vi "Scanner_Ansteuerung_Prepare_Puls_Sequence.vi"(11 "cluster":T1) -> (0 "Sync-Pulse-Array":bool[](array[boolean]), 1 "Power-Array":dbl[][][](array[numeric]), 3 "Clock-Array":i32[](array[numeric]))   [LabVIEW 2009]
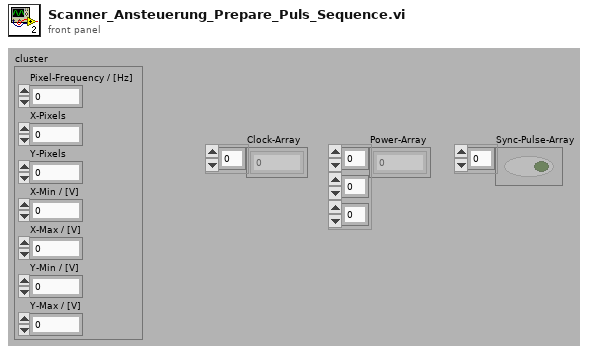
[diagram p1: front panel]
types:
  T1 = cluster{"Pixel-Frequency / [Hz]":dbl, "X-Pixels":u32, "Y-Pixels":u32, "X-Min / [V]":dbl, "X-Max / [V]":dbl, "Y-Min / [V]":dbl, "Y-Max / [V]":dbl}
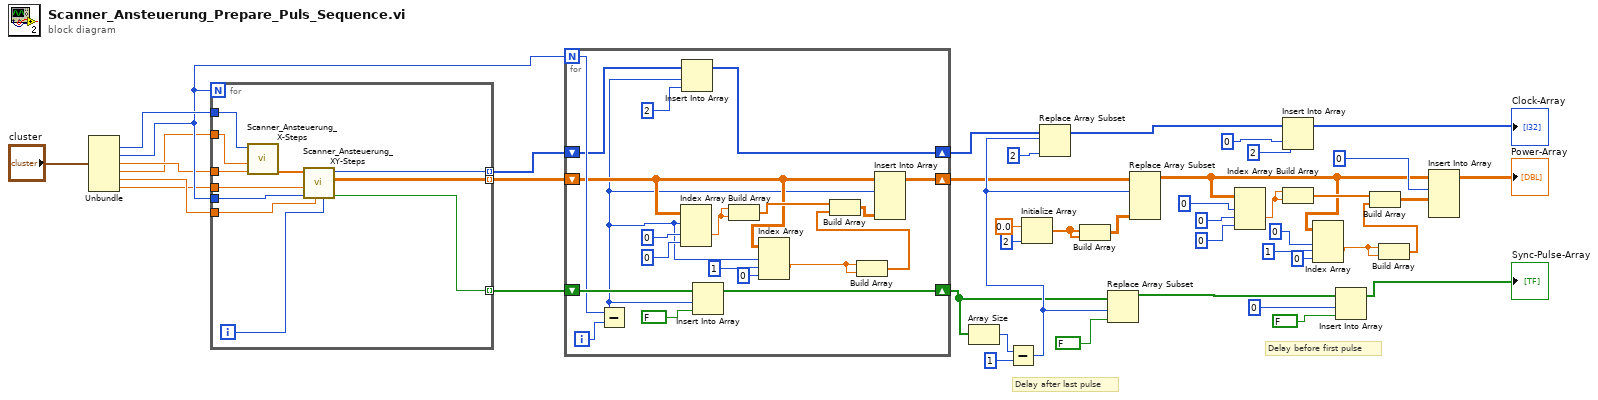
[diagram p0: block diagram]
diagram:
  # "Delay before first pulse"
  # "Delay after last pulse"
  n1 = Unbundle("cluster") -> ("X-Pixels"=w6:u32, "Y-Pixels"=w5:u32, "X-Min / [V]"=w4:dbl, "X-Max / [V]"=w3:dbl, "Y-Min / [V]"=w2:dbl, "Y-Max / [V]"=w1:dbl)  [unwired: 1 out]
  n2 = for {
    N: w5 -> [_]
    tunnel: w2 -> [w55]
    tunnel: w4 -> [w54]
    tunnel: w6 -> [w53]
    tunnel: w3 -> [w52]
    tunnel: w1 -> [w51]
    tunnel: w5 -> [w50]
    tunnel: [w49] -> w9 mode=indexing
    tunnel: [w47] -> w8 mode=indexing
    tunnel: [w46] -> w10 mode=indexing
    i -> [w45]
    n3 = call "Scanner_Ansteuerung_X-Steps.vi"("X-Min / [V]"=w54, "X-Max / [V]"=w52, "X-Pixels"=w53) -> ("X-Array out"=w48:dbl[])  [unwired: 8 out]
    n4 = call "Scanner_Ansteuerung_XY-Steps.vi"("Loop-Count for Y"=w45, "Y-Min / [V]"=w55, "Y-Pixels"=w50, "Y-Max / [V]"=w51, "X-Array in"=w48) -> ("x < y?"=w46:bool, "XY-Array out"=w49:dbl[][], "Samples per channel"=w47:i32)  [unwired: 2 in, 2 out]
  }
  n5 = for {
    N: w5 -> [w73]
    shift-right: [w75] -> w19
    shift-left: w10 -> [w74]
    shift-right: [w69] -> w11
    shift-left: w8 -> [w70]
    shift-right: [w67] -> w18
    shift-left: w9 -> [w59]
    i -> [w72]
    n6 = Subtract(x=w73, y=w72) -> (x-y=w56:i32)
    n7 = Index Array(array=w59, index (dim 0)=w56, index (dim 1)=0 ("disabled index (row)"), index (dim 2)=0 ("disabled index (col)")) -> (element=w61:dbl)
    n8 = Insert Into Array(array=w70, index=w56, new element=2 ("new element/subarray")) -> (w69:i32[])
    n9 = Insert Into Array(array=w74, index=w56, new element=FALSE ("new element/subarray")) -> (w75:bool[])
    n10 = Build Array(w61, w61) -> (w64:dbl[])
    n11 = Index Array(array=w59, index (dim 0)=w56, index (dim 1)=1 ("disabled index (row)"), index (dim 2)=0 ("disabled index (col)")) -> (element=w60:dbl)
    n12 = Build Array(w60, w60) -> (w63:dbl[])
    n13 = Build Array(w64, w63) -> (w62:dbl[][])
    n14 = Insert Into Array(array=w59, index (dim 0)=w56, new element=w62) -> (w67:dbl[][][])  [unwired: 2 in]
  }
  n15 = Array Size(array=w19) -> (size(s)=w20:i32)
  n16 = Subtract(x=w20, y=1) -> (x-y=w21:i32)
  n17 = Initialize Array(0.0 ("element"), 2 ("dimension size")) -> (w16:dbl[])
  n18 = Replace Array Subset(array=w11, new element=2 ("new element/subarray"), index=w21) -> (w41:i32[])
  n19 = Build Array(w16, w16) -> (w17:dbl[][])
  n20 = Replace Array Subset(array=w19, new element=FALSE ("new element/subarray"), index=w21) -> (w38:bool[])
  n21 = Replace Array Subset(array=w18, new element=w17, index (dim 0)=w21) -> (w29:dbl[][][])  [unwired: 2 in]
  n22 = Index Array(array=w29, index (dim 0)=0 ("disabled index (row)"), index (dim 1)=0 ("disabled index (row)"), index (dim 2)=0 ("disabled index (col)")) -> (element=w25:dbl)
  n23 = Insert Into Array(array=w41, index=0, new element=2 ("new element/subarray")) -> (→"Clock-Array":i32[])
  n24 = Build Array(w25, w25) -> (w35:dbl[])
  n25 = Index Array(array=w29, index (dim 0)=0 ("disabled index (page)"), index (dim 1)=1 ("disabled index (row)"), index (dim 2)=0 ("disabled index (col)")) -> (element=w26:dbl)
  n26 = Insert Into Array(array=w38, index=0, new element=FALSE ("new element/subarray")) -> (→"Sync-Pulse-Array":bool[])
  n27 = Build Array(w26, w26) -> (w36:dbl[])
  n28 = Build Array(w35, w36) -> (w34:dbl[][])
  n29 = Insert Into Array(array=w29, index (dim 0)=0 ("index (page)"), new element=w34) -> (→"Power-Array":dbl[][][])  [unwired: 2 in]
